vi "Create Serial Input Channel I2C IO x8.vi"() -> (4 "serial input channel i2c io x8":T2)   [LabVIEW 2023, in "GettingStarted_Acq_Tap_148X_FPGA.lvlib"]
uses:
  GettingStarted_Acq_Tap_148X_FPGA.lvlib
  Common/Types/I2C IO.ctl
  Common/GettingStarted_Common_148X_FPGA.lvlib
  <instrlib>/_niInstr/Basic Elements/v1/FPGA/niInstr Basic Elements v1 FPGA.lvlib
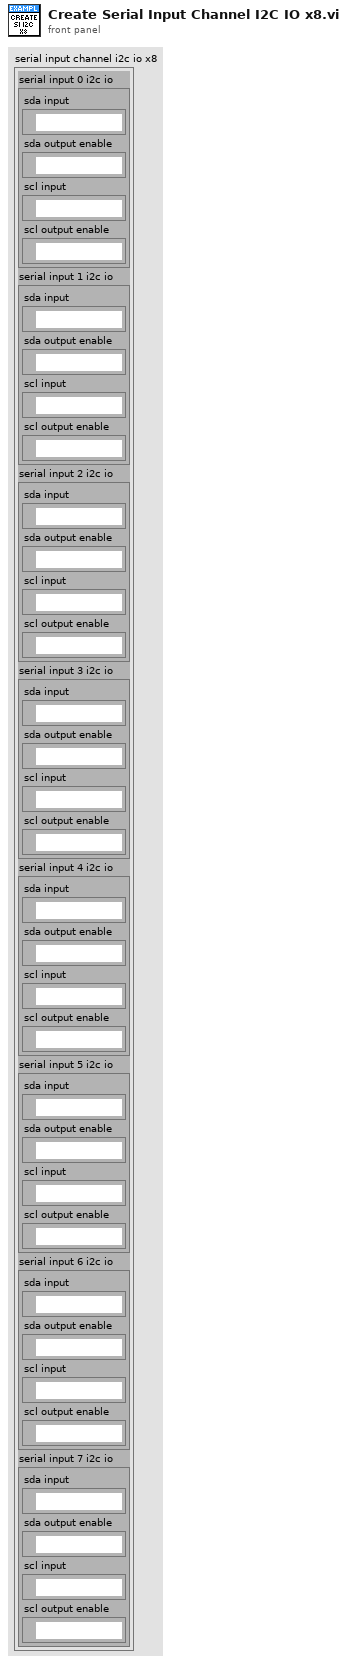
[diagram p1: front panel]
types:
  T1 = typedef "GettingStarted_Common_148X_FPGA.lvlib/I2C IO.ctl" = cluster{"sda input":refnum<k21>, "sda output enable":refnum<k21>, "scl input":refnum<k21>, "scl output enable":refnum<k21>}
  T2 = cluster{"serial input 0 i2c io":T1, "serial input 1 i2c io":T1, "serial input 2 i2c io":T1, "serial input 3 i2c io":T1, "serial input 4 i2c io":T1, "serial input 5 i2c io":T1, "serial input 6 i2c io":T1, "serial input 7 i2c io":T1}
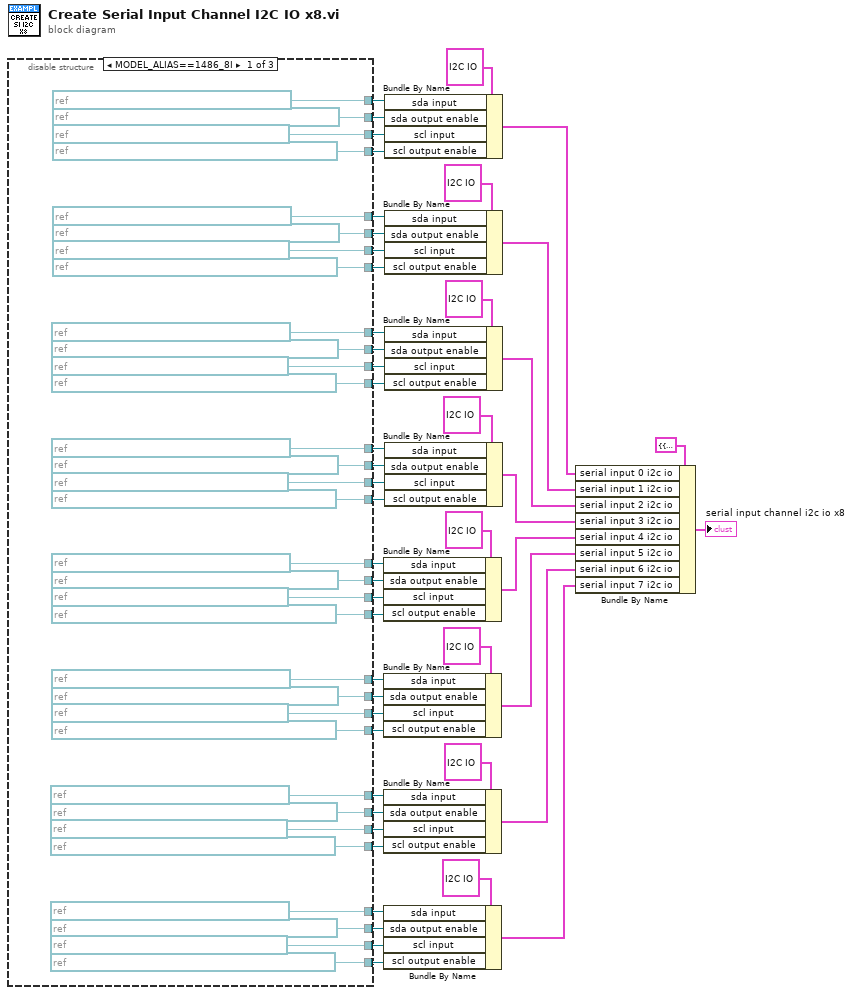
[diagram p0: block diagram]
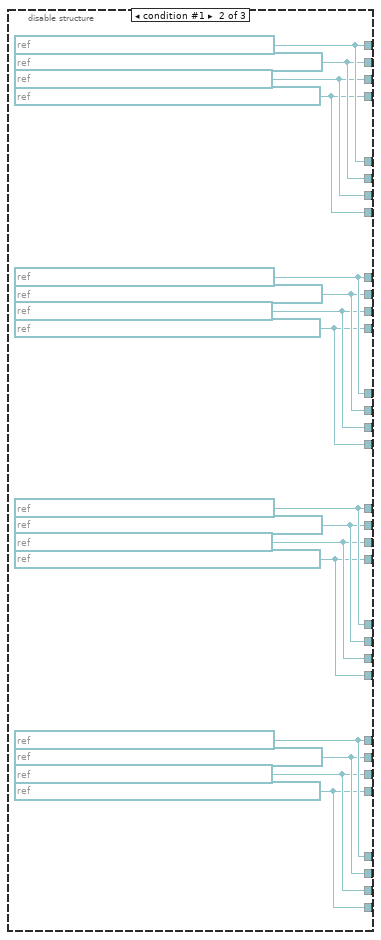
[diagram p2: hidden frame]
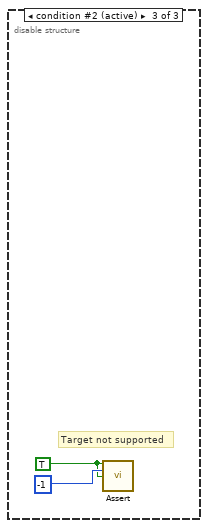
[diagram p3: hidden frame]
diagram:
  n1 = disable-structure shown="MODEL_ALIAS==1486_8I" {
    disable-tunnel: [refnum<k21> "IO Socket\\SI 2 Deserializer I2C SCL Output Enable" ("scl output enable") w91 _] -> w45
    disable-tunnel: [refnum<k21> "IO Socket\\SI 2 Deserializer I2C SCL Input" ("scl input") w92 _] -> w44
    disable-tunnel: [refnum<k21> "IO Socket\\SI 2 Deserializer I2C SDA Output Enable" ("sda output enable") w93 _] -> w43
    disable-tunnel: [refnum<k21> "IO Socket\\SI 2 Deserializer I2C SDA Input" ("sda input") w94 _] -> w42
    disable-tunnel: [refnum<k21> "IO Socket\\SI 3 Deserializer I2C SDA Input" ("sda input") w94 _] -> w39
    disable-tunnel: [refnum<k21> "IO Socket\\SI 3 Deserializer I2C SDA Output Enable" ("sda output enable") w93 _] -> w38
    disable-tunnel: [refnum<k21> "IO Socket\\SI 3 Deserializer I2C SCL Input" ("scl input") w92 _] -> w37
    disable-tunnel: [refnum<k21> "IO Socket\\SI 3 Deserializer I2C SCL Output Enable" ("scl output enable") w91 _] -> w36
    disable-tunnel: [refnum<k21> "IO Socket\\SI 1 Deserializer I2C SCL Output Enable" ("scl output enable") w95 _] -> w35
    disable-tunnel: [refnum<k21> "IO Socket\\SI 1 Deserializer I2C SCL Input" ("scl input") w96 _] -> w34
    disable-tunnel: [refnum<k21> "IO Socket\\SI 1 Deserializer I2C SDA Output Enable" ("sda output enable") w97 _] -> w33
    disable-tunnel: [refnum<k21> "IO Socket\\SI 1 Deserializer I2C SDA Input" ("sda input") w98 _] -> w32
    disable-tunnel: [refnum<k21> "IO Socket\\SI 0 Deserializer I2C SDA Input" ("sda input") w98 _] -> w29
    disable-tunnel: [refnum<k21> "IO Socket\\SI 0 Deserializer I2C SDA Output Enable" ("sda output enable") w97 _] -> w28
    disable-tunnel: [refnum<k21> "IO Socket\\SI 0 Deserializer I2C SCL Input" ("scl input") w96 _] -> w27
    disable-tunnel: [refnum<k21> "IO Socket\\SI 0 Deserializer I2C SCL Output Enable" ("scl output enable") w95 _] -> w26
    disable-tunnel: [refnum<k21> "IO Socket\\SI 4 Deserializer I2C SCL Output Enable" ("scl output enable") w87 _] -> w24
    disable-tunnel: [refnum<k21> "IO Socket\\SI 4 Deserializer I2C SCL Input" ("scl input") w88 _] -> w23
    disable-tunnel: [refnum<k21> "IO Socket\\SI 4 Deserializer I2C SDA Output Enable" ("sda output enable") w89 _] -> w22
    disable-tunnel: [refnum<k21> "IO Socket\\SI 4 Deserializer I2C SDA Input" ("sda input") w90 _] -> w21
    disable-tunnel: [refnum<k21> "IO Socket\\SI 5 Deserializer I2C SDA Input" ("sda input") w90 _] -> w18
    disable-tunnel: [refnum<k21> "IO Socket\\SI 5 Deserializer I2C SDA Output Enable" ("sda output enable") w89 _] -> w17
    disable-tunnel: [refnum<k21> "IO Socket\\SI 5 Deserializer I2C SCL Input" ("scl input") w88 _] -> w16
    disable-tunnel: [refnum<k21> "IO Socket\\SI 5 Deserializer I2C SCL Output Enable" ("scl output enable") w87 _] -> w15
    disable-tunnel: [refnum<k21> "IO Socket\\SI 7 Deserializer I2C SCL Output Enable" ("scl output enable") w83 _] -> w14
    disable-tunnel: [refnum<k21> "IO Socket\\SI 7 Deserializer I2C SCL Input" ("scl input") w84 _] -> w13
    disable-tunnel: [refnum<k21> "IO Socket\\SI 7 Deserializer I2C SDA Output Enable" ("sda output enable") w85 _] -> w12
    disable-tunnel: [refnum<k21> "IO Socket\\SI 7 Deserializer I2C SDA Input" ("sda input") w86 _] -> w11
    disable-tunnel: [refnum<k21> "IO Socket\\SI 6 Deserializer I2C SDA Input" ("sda input") w86 _] -> w8
    disable-tunnel: [refnum<k21> "IO Socket\\SI 6 Deserializer I2C SDA Output Enable" ("sda output enable") w85 _] -> w7
    disable-tunnel: [refnum<k21> "IO Socket\\SI 6 Deserializer I2C SCL Input" ("scl input") w84 _] -> w6
    disable-tunnel: [refnum<k21> "IO Socket\\SI 6 Deserializer I2C SCL Output Enable" ("scl output enable") w83 _] -> w5
    frame condition #0 {
    }
    frame condition #1 {
      w83 = refnum<k21> "IO Socket\\SI 6 SI 7 Deserializer I2C SCL Output Enable" ("scl output enable")
      w84 = refnum<k21> "IO Socket\\SI 6 SI 7 Deserializer I2C SCL Input" ("scl input")
      w85 = refnum<k21> "IO Socket\\SI 6 SI 7 Deserializer I2C SDA Output Enable" ("sda output enable")
      w86 = refnum<k21> "IO Socket\\SI 6 SI 7 Deserializer I2C SDA Input" ("sda input")
      w87 = refnum<k21> "IO Socket\\SI 4 SI 5 Deserializer I2C SCL Output Enable" ("scl output enable")
      w88 = refnum<k21> "IO Socket\\SI 4 SI 5 Deserializer I2C SCL Input" ("scl input")
      w89 = refnum<k21> "IO Socket\\SI 4 SI 5 Deserializer I2C SDA Output Enable" ("sda output enable")
      w90 = refnum<k21> "IO Socket\\SI 4 SI 5 Deserializer I2C SDA Input" ("sda input")
      w91 = refnum<k21> "IO Socket\\SI 2 SI 3 Deserializer I2C SCL Output Enable" ("scl output enable")
      w92 = refnum<k21> "IO Socket\\SI 2 SI 3 Deserializer I2C SCL Input" ("scl input")
      w93 = refnum<k21> "IO Socket\\SI 2 SI 3 Deserializer I2C SDA Output Enable" ("sda output enable")
      w94 = refnum<k21> "IO Socket\\SI 2 SI 3 Deserializer I2C SDA Input" ("sda input")
      w95 = refnum<k21> "IO Socket\\SI 0 SI 1 Deserializer I2C SCL Output Enable" ("scl output enable")
      w96 = refnum<k21> "IO Socket\\SI 0 SI 1 Deserializer I2C SCL Input" ("scl input")
      w97 = refnum<k21> "IO Socket\\SI 0 SI 1 Deserializer I2C SDA Output Enable" ("sda output enable")
      w98 = refnum<k21> "IO Socket\\SI 0 SI 1 Deserializer I2C SDA Input" ("sda input")
    }
    frame condition #2 (active) {
      w99 = TRUE ("assert")
      # "Target not supported"
      n2 = call <instrlib>:"Assert.vi"("assert"=w99, "error code"=-1, "enable show error"=w99) -> ()  [unwired: 13 in]
    }
  }
  n3 = Bundle By Name(cluster=T1 {"sda input"="IO Socket\\SI 0 Deserializer I2C SDA Input", "sda output enable"="IO Socket\\SI 0 Deserializer I2C SDA Output Enable", "scl input"="IO Socket\\SI 0 Deserializer I2C SCL Input", "scl output enable"="IO Socket\\SI 0 Deserializer I2C SCL Output Enable"}, "sda input"=w21, "sda output enable"=w22, "scl input"=w23, "scl output enable"=w24) -> (w4:T1)
  n4 = Bundle By Name(cluster=T1 {"sda input"="IO Socket\\SI 0 Deserializer I2C SDA Input", "sda output enable"="IO Socket\\SI 0 Deserializer I2C SDA Output Enable", "scl input"="IO Socket\\SI 0 Deserializer I2C SCL Input", "scl output enable"="IO Socket\\SI 0 Deserializer I2C SCL Output Enable"}, "sda input"=w18, "sda output enable"=w17, "scl input"=w16, "scl output enable"=w15) -> (w3:T1)
  n5 = Bundle By Name(cluster=T1 {"sda input"="IO Socket\\SI 0 Deserializer I2C SDA Input", "sda output enable"="IO Socket\\SI 0 Deserializer I2C SDA Output Enable", "scl input"="IO Socket\\SI 0 Deserializer I2C SCL Input", "scl output enable"="IO Socket\\SI 0 Deserializer I2C SCL Output Enable"}, "sda input"=w8, "sda output enable"=w7, "scl input"=w6, "scl output enable"=w5) -> (w2:T1)
  n6 = Bundle By Name(cluster=T1 {"sda input"="IO Socket\\SI 0 Deserializer I2C SDA Input", "sda output enable"="IO Socket\\SI 0 Deserializer I2C SDA Output Enable", "scl input"="IO Socket\\SI 0 Deserializer I2C SCL Input", "scl output enable"="IO Socket\\SI 0 Deserializer I2C SCL Output Enable"}, "sda input"=w11, "sda output enable"=w12, "scl input"=w13, "scl output enable"=w14) -> (w1:T1)
  n7 = Bundle By Name(cluster=T1 {"sda input"="IO Socket\\SI 0 Deserializer I2C SDA Input", "sda output enable"="IO Socket\\SI 0 Deserializer I2C SDA Output Enable", "scl input"="IO Socket\\SI 0 Deserializer I2C SCL Input", "scl output enable"="IO Socket\\SI 0 Deserializer I2C SCL Output Enable"}, "sda input"=w29, "sda output enable"=w28, "scl input"=w27, "scl output enable"=w26) -> (w47:T1)
  n8 = Bundle By Name(cluster=T1 {"sda input"="IO Socket\\SI 0 Deserializer I2C SDA Input", "sda output enable"="IO Socket\\SI 0 Deserializer I2C SDA Output Enable", "scl input"="IO Socket\\SI 0 Deserializer I2C SCL Input", "scl output enable"="IO Socket\\SI 0 Deserializer I2C SCL Output Enable"}, "sda input"=w32, "sda output enable"=w33, "scl input"=w34, "scl output enable"=w35) -> (w48:T1)
  n9 = Bundle By Name(cluster=T1 {"sda input"="IO Socket\\SI 0 Deserializer I2C SDA Input", "sda output enable"="IO Socket\\SI 0 Deserializer I2C SDA Output Enable", "scl input"="IO Socket\\SI 0 Deserializer I2C SCL Input", "scl output enable"="IO Socket\\SI 0 Deserializer I2C SCL Output Enable"}, "sda input"=w42, "sda output enable"=w43, "scl input"=w44, "scl output enable"=w45) -> (w49:T1)
  n10 = Bundle By Name(cluster=T1 {"sda input"="IO Socket\\SI 0 Deserializer I2C SDA Input", "sda output enable"="IO Socket\\SI 0 Deserializer I2C SDA Output Enable", "scl input"="IO Socket\\SI 0 Deserializer I2C SCL Input", "scl output enable"="IO Socket\\SI 0 Deserializer I2C SCL Output Enable"}, "sda input"=w39, "sda output enable"=w38, "scl input"=w37, "scl output enable"=w36) -> (w50:T1)
  n11 = Bundle By Name(cluster=T2 {"serial input 0 i2c io"={"sda input"="IO Socket\\SI 0 Deserializer I2C SDA Input", "sda output enable"="IO Socket\\SI 0 Deserializer I2C SDA Output Enable", "scl input"="IO Socket\\SI 0 Deserializer I2C SCL Input", "scl output enable"="IO Socket\\SI 0 Deserializer I2C SCL Output Enable"}, "serial input 1 i2c io"={"sda input"="IO Socket\\SI 0 Deserializer I2C SDA Input", "sda output enable"="IO Socket\\SI 0 Deserializer I2C SDA Output Enable", "scl input"="IO Socket\\SI 0 Deserializer I2C SCL Input", "scl output enable"="IO Socket\\SI 0 Deserializer I2C SCL Output Enable"}, "serial input 2 i2c io"={"sda input"="IO Socket\\SI 0 Deserializer I2C SDA Input", "sda output enable"="IO Socket\\SI 0 Deserializer I2C SDA Output Enable", "scl input"="IO Socket\\SI 0 Deserializer I2C SCL Input", "scl output enable"="IO Socket\\SI 0 Deserializer I2C SCL Output Enable"}, "serial input 3 i2c io"={"sda input"="IO Socket\\SI 0 Deserializer I2C SDA Input", "sda output enable"="IO Socket\\SI 0 Deserializer I2C SDA Output Enable", "scl input"="IO Socket\\SI 0 Deserializer I2C SCL Input", "scl output enable"="IO Socket\\SI 0 Deserializer I2C SCL Output Enable"}, "serial input 4 i2c io"={"sda input"="IO Socket\\SI 0 Deserializer I2C SDA Input", "sda output enable"="IO Socket\\SI 0 Deserializer I2C SDA Output Enable", "scl input"="IO Socket\\SI 0 Deserializer I2C SCL Input", "scl output enable"="IO Socket\\SI 0 Deserializer I2C SCL Output Enable"}, "serial input 5 i2c io"={"sda input"="IO Socket\\SI 0 Deserializer I2C SDA Input", "sda output enable"="IO Socket\\SI 0 Deserializer I2C SDA Output Enable", "scl input"="IO Socket\\SI 0 Deserializer I2C SCL Input", "scl output enable"="IO Socket\\SI 0 Deserializer I2C SCL Output Enable"}, "serial input 6 i2c io"={"sda input"="IO Socket\\SI 0 Deserializer I2C SDA Input", "sda output enable"="IO Socket\\SI 0 Deserializer I2C SDA Output Enable", "scl input"="IO Socket\\SI 0 Deserializer I2C SCL Input", "scl output enable"="IO Socket\\SI 0 Deserializer I2C SCL Output Enable"}, "serial input 7 i2c io"={"sda input"="IO Socket\\SI 0 Deserializer I2C SDA Input", "sda output enable"="IO Socket\\SI 0 Deserializer I2C SDA Output Enable", "scl input"="IO Socket\\SI 0 Deserializer I2C SCL Input", "scl output enable"="IO Socket\\SI 0 Deserializer I2C SCL Output Enable"}} ("serial input channel i2c io x4"), "serial input 0 i2c io"=w47, "serial input 1 i2c io"=w48, "serial input 2 i2c io"=w49, "serial input 3 i2c io"=w50, "serial input 4 i2c io"=w4, "serial input 5 i2c io"=w3, "serial input 6 i2c io"=w2, "serial input 7 i2c io"=w1) -> (→"serial input channel i2c io x8":T2)
